vi "Interpolator.vi"(10 "array of numbers or points":cluster{"x":dbl, "y":dbl}[](array[cluster]), 11 "Temperature":dbl) -> (3 "interpolation value":dbl)   [LabVIEW 2013]
uses:
  <vilib>/Analysis/NI_AALPro.lvlib
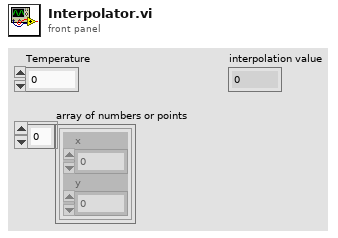
[diagram p1: front panel]
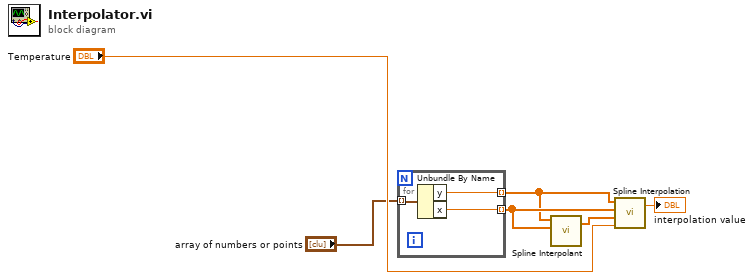
[diagram p0: block diagram]
diagram:
  n1 = for {
    tunnel: "array of numbers or points" -> [w9] mode=indexing
    tunnel: [w8] -> w3 mode=indexing
    tunnel: [w7] -> w4 mode=indexing
    n2 = Unbundle By Name(w9) -> ("y"=w8:dbl, "x"=w7:dbl)
  }
  n3 = call <vilib>:"Spline Interpolant.vi"("X"=w4, "Y"=w3) -> ("Interpolant"=w2:dbl[])  [unwired: 2 in, 1 out]
  n4 = call <vilib>:"Spline Interpolation.vi"("x value"="Temperature", "Interpolant"=w2, "X"=w4, "Y"=w3) -> ("interpolation value"=→"interpolation value":dbl)  [unwired: 1 out]
